vi "MGCC_MdlMgmt_Loads.vi"() -> ()   [LabVIEW 2016]
doc: "This VI is designed to initize the SHE215 model with loads (2D double array)."
uses:
  <vilib>/imath/engines/lvmath2/RunTimeEngine/NodeEndStatement/NIMS_NodeEndStatement_Output.vi
  <instcachedir>/0/NIMS_NodeEndStatement_Output_53EC0D466D134D7ABD903AC30B43404B.lvgen/NIMS_NodeEndStatement_Output_53EC0D466D134D7ABD903AC30B43404B_002.vi
  <vilib>/imath/engines/lvmath2/RunTimeEngine/ErrorHandling/NIMS_Finalize Error.vi
panel:
  out "array":dbl[][](array[numeric])
  out "text":string
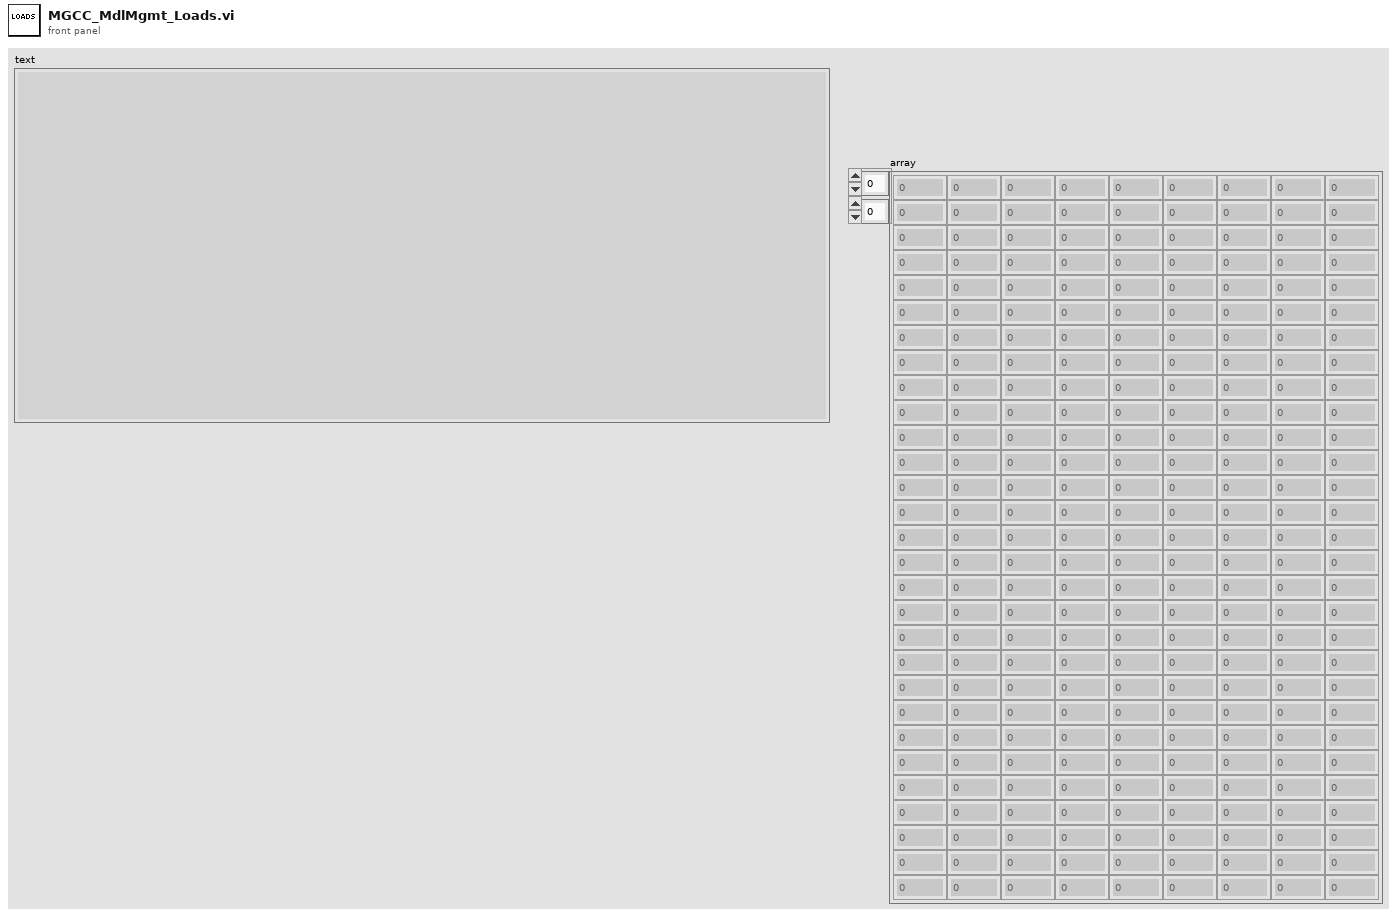
[diagram p1: front panel]
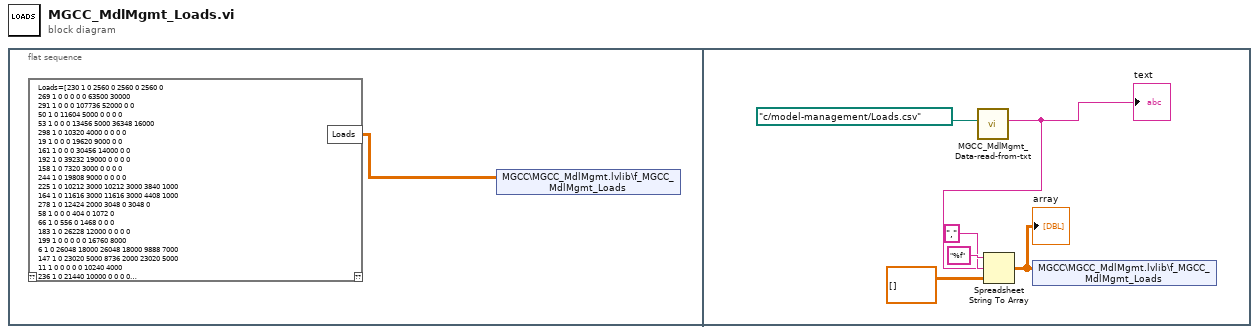
[diagram p0: block diagram]
diagram:
  n1 = flat-sequence {
    frame #0 {
      n2 = mathscript code="Loads=[230\t1\t0\t2560\t0\t2560\t0\t2560\t0\n269\t1\t0\t0\t0\t0\t0\t63500\t30000\n291\t1\t0\t0\t0\t107736\t52000\t0\t0\n50\t1\t0\t11604\t5000\t0\t0\t0\t0\n53\t1\t0\t0\t0\t13456\t5000\t36348\t16000\n298\t1\t0\t10320\t4000\t0\t0\t0\t0\n19\t1\t0\t0\t0\t19620\t9000\t0\t0\n161\t1\t0\t0\t0\t30456\t14000\t0\t0\n192\t1\t0\t39232\t19000\t0\t0\t0\t0\n158\t1\t0\t7320\t3000\t0\t0\t0\t0\n244\t1\t0\t19808\t9000\t0\t0\t0\t0\n225\t1\t0\t10212\t3000\t10212\t3000\t3840\t1000\n164\t1\t0\t11616\t3000\t11616\t3000\t4408\t1000\n278\t1\t0\t12424\t2000\t3048\t0\t3048\t0\n58\t1\t0\t0\t0\t404\t0\t1072\t0\n66\t1\t0\t556\t0\t1468\t0\t0\t0\n183\t1\t0\t26228\t12000\t0\t0\t0\t0\n199\t1\t0\t0\t0\t0\t0\t16760\t8000\n6\t1\t0\t26048\t18000\t26048\t18000\t9888\t7000\n147\t1\t0\t23020\t5000\t8736\t2000\t23020\t5000\n11\t1\t0\t0\t0\t0\t0\t10240\t4000\n236\t1\t0\t21440\t10000\t0\t0\t0\t0\n292\t1\t0\t0\t0\t7232\t3000\t0\t0\n163\t1\t0\t80516\t39000\t0\t0\t0\t0\n174\t1\t0\t33692\t16000\t0\t0\t0\t0\n133\t1\t0\t6412\t1000\t22208\t6000\t22208\t6000\n152\t1\t0\t1464\t0\t0\t0\t0\t0\n253\t1\t0\t10128\t5000\t26680\t13000\t26680\t13000\n218\t1\t0\t0\t0\t44332\t21000\t0\t0\n231\t1\t0\t0\t0\t0\t0\t47604\t23000\n61\t1\t0\t0\t0\t3384\t2000\t8948\t6000\n193\t1\t0\t0\t0\t60444\t29000\t0\t0\n207\t1\t0\t6444\t4000\t6444\t4000\t2404\t1000\n277\t1\t0\t32972\t15000\t0\t0\t0\t0\n57\t1\t0\t10560\t1000\t10560\t1000\t4008\t0\n17\t1\t0\t0\t0\t22604\t10000\t0\t0\n29\t1\t0\t0\t0\t0\t0\t12540\t6000\n22\t1\t0\t10916\t5000\t0\t0\t1732\t0\n166\t1\t0\t0\t0\t0\t0\t16996\t8000\n279\t1\t0\t22396\t3000\t22396\t3000\t22396\t3000\n224\t1\t0\t2932\t1000\t2932\t1000\t2932\t1000\n14\t1\t0\t2436\t0\t2436\t0\t924\t0\n123\t1\t0\t0\t0\t7226.66800000000\t5000\t7226.66800000000\t5000\n30\t1\t0\t0\t0\t12864\t6000\t0\t0\n280\t1\t0\t0\t0\t22808\t11000\t0\t0\n71\t1\t0\t0\t0\t0\t0\t17616\t8000\n167\t1\t0\t0\t0\t19296\t9000\t0\t0\n245\t1\t0\t0\t0\t0\t0\t26548\t12000\n246\t1\t0\t51136\t24000\t0\t0\t0\t0\n82\t1\t0\t2000\t1000\t2000\t1000\t2000\t1000\n2\t1\t0\t8008.00000000000\t2000\t8008.00000000000\t2000\t8008.00000000000\t2000\n266\t1\t0\t15176\t2000\t15176\t2000\t5720\t0\n191\t1\t0\t0\t0\t4188\t2000\t0\t0\n281\t1\t0\t11520\t3000\t11520\t3000\t11520\t3000\n222\t1\t0\t27944\t4000\t27944\t4000\t27944\t4000\n299\t1\t0\t0\t0\t0\t0\t57232\t27000\n142\t1\t0\t0\t0\t0\t0\t39868\t19000\n52\t1\t0\t0\t0\t0\t0\t34656\t16000\n295\t1\t0\t37948\t18000\t0\t0\t0\t0\n77\t1\t0\t9404\t2000\t24780\t7000\t24780\t7000\n284\t1\t0\t0\t0\t876\t0\t2312\t0\n28\t1\t0\t0\t0\t0\t0\t12292\t5000\n188\t1\t0\t19256\t9000\t0\t0\t0\t0\n78\t1\t0\t746.668000000000\t0\t746.668000000000\t0\t746.668000000000\t0\n223\t1\t0\t0\t0\t0\t0\t42192\t20000\n39\t1\t0\t17600\t8000\t0\t0\t0\t0\n283\t1\t0\t32996\t14000\t32996\t14000\t32996\t14000\n81\t1\t0\t0\t0\t0\t0\t32980\t15000\n238\t1\t0\t43344\t21000\t0\t0\t0\t0\n153\t1\t0\t9200\t4000\t9200\t4000\t9200\t4000\n160\t1\t0\t900\t0\t0\t0\t0\t0\n184\t1\t0\t0\t0\t0\t0\t20420\t9000\n293\t1\t0\t10452\t4000\t10452\t4000\t10452\t4000\n141\t1\t0\t4320\t2000\t0\t0\t0\t0\n5\t1\t0\t0\t0\t0\t0\t10212\t4000\n262\t1\t0\t4360\t0\t4360\t0\t4360\t0\n237\t1\t0\t0\t0\t8560\t4000\t0\t0\n121\t1\t0\t0\t0\t43704\t21000\t0\t0\n228\t1\t0\t45936\t22000\t7320\t3000\t7320\t3000\n101\t1\t0\t0\t0\t0\t0\t63344\t30000\n255\t1\t0\t0\t0\t0\t0\t59820\t28000\n104\t1\t0\t9944\t3000\t0\t0\t3760\t1000\n210\t1\t0\t27556\t13000\t0\t0\t0\t0\n263\t1\t0\t26292\t9000\t26292\t9000\t6440\t1000\n221\t1\t0\t22576\t10000\t22576\t10000\t420\t0\n33\t1\t0\t1324\t0\t1324\t0\t1324\t0\n242\t1\t0\t1068\t0\t1068\t0\t1068\t0\n235\t1\t0\t17704\t1000\t17704\t1000\t17704\t1000\n240\t1\t0\t0\t0\t0\t0\t18944\t9000\n226\t1\t0\t20084\t3000\t20084\t3000\t20084\t3000\n270\t1\t0\t7056\t3000\t156\t0\t0\t0\n72\t1\t0\t14688\t7000\t0\t0\t0\t0\n258\t1\t0\t0\t0\t0\t0\t50752\t24000\n75\t1\t0\t928\t0\t0\t0\t0\t0\n243\t1\t0\t0\t0\t0\t0\t16256\t7000\n286\t1\t0\t3840\t1000\t0\t0\t0\t0\n256\t1\t0\t9332\t2000\t9332\t2000\t9332\t2000\n48\t1\t0\t16212\t3000\t16212\t3000\t16212\t3000\n135\t1\t0\t22012\t10000\t0\t0\t0\t0\n143\t1\t0\t640\t0\t1688\t1000\t1688\t1000\n190\t1\t0\t0\t0\t0\t0\t8088.00000000000\t3000\n220\t1\t0\t0\t0\t0\t0\t2048\t0\n124\t1\t0\t0\t0\t5192\t2000\t0\t0\n95\t1\t0\t640\t0\t1688\t1000\t1688\t1000\n211\t1\t0\t0\t0\t10860\t5000\t0\t0\n213\t1\t0\t19744\t9000\t0\t0\t0\t0\n289\t1\t0\t13120\t4000\t13120\t4000\t13120\t4000\n296\t1\t0\t0\t0\t0\t0\t26912\t13000\n185\t1\t0\t4716\t1000\t4716\t1000\t1792\t0\n45\t1\t0\t1920\t2000\t1920\t2000\t1920\t2000\n249\t1\t0\t0\t0\t2960\t0\t7960\t1000\n271\t1\t0\t15572\t3000\t15572\t3000\t15572\t3000\n54\t1\t0\t11652\t5000\t0\t0\t0\t0\n180\t1\t0\t0\t0\t0\t0\t57236\t27000\n251\t1\t0\t36360\t17000\t0\t0\t0\t0\n265\t1\t0\t83860\t14000\t83860\t14000\t83860\t14000\n227\t1\t0\t2432\t1000\t9216\t4000\t9216\t4000\n282\t1\t0\t9064\t3000\t9064\t3000\t9064\t3000\n259\t1\t0\t0\t0\t3908\t1000\t0\t0\n51\t1\t0\t22808\t11000\t0\t0\t0\t0\n294\t1\t0\t16852\t7000\t16852\t7000\t16852\t7000\n268\t1\t0\t0\t0\t0\t0\t33892\t16000\n115\t1\t0\t0\t0\t76\t0\t0\t0\n288\t1\t0\t103456\t33000\t103456\t33000\t103456\t33000\n155\t1\t0\t4864\t2000\t0\t0\t0\t0\n287\t1\t0\t62856\t30000\t0\t0\t0\t0\n70\t1\t0\t0\t0\t33960\t16000\t0\t0\n168\t1\t0\t3632\t0\t3632\t0\t17744\t4000\n241\t1\t0\t852\t0\t0\t0\t0\t0\n165\t1\t0\t0\t0\t10044\t4000\t0\t0\n254\t1\t0\t0\t0\t616\t0\t0\t0\n234\t1\t0\t1600\t0\t1600\t0\t1600\t0\n195\t1\t0\t0\t0\t34356\t16000\t0\t0\n47\t1\t0\t0\t0\t0\t0\t408\t0\n10\t1\t0\t0\t0\t5316\t2000\t14056\t5000\n208\t1\t0\t12160\t5000\t0\t0\t0\t0\n202\t1\t0\t0\t0\t0\t0\t31764\t15000\n179\t1\t0\t0\t0\t7380\t0\t28308\t7000\n267\t1\t0\t76364\t0\t76364\t0\t76364\t0\n248\t1\t0\t3732\t1000\t3732\t1000\t3732\t1000\n276\t1\t0\t21384\t3000\t21384\t3000\t21384\t3000\n297\t1\t0\t12888\t2000\t12888\t2000\t12888\t2000\n216\t1\t0\t720\t0\t720\t0\t720\t0\n219\t1\t0\t0\t0\t0\t0\t67472\t32000\n9\t1\t0\t0\t0\t21872\t9000\t2452\t0\n114\t1\t0\t13568\t0\t5132\t0\t0\t0\n84\t1\t0\t6480\t3000\t0\t0\t0\t0\n131\t1\t0\t0\t0\t0\t0\t11040\t5000];"() -> ("Loads"=w1:dbl[][])  [unwired: 1 in, 1 out]
      n3 = shared-variable "MGCC\\MGCC_MdlMgmt.lvlib\\f_MGCC_MdlMgmt_Loads"(w1) -> ()  [unwired: 1 in, 1 out]
    }
    frame #1 {
      n4 = call "MGCC_MdlMgmt_Data-read-from-txt.vi"("file path (use dialog)"=path "c:/model-management/Loads.csv") -> ("text"=w15:string)  [unwired: 10 in]
      "text" <- w15
      n5 = Spreadsheet String To Array(delimiter (Tab)=",", format string="%f", spreadsheet string=w15, array type (2D Dbl)=dbl[][] []) -> (array=w16:dbl[][])
      "array" <- w16
      n6 = shared-variable "MGCC\\MGCC_MdlMgmt.lvlib\\f_MGCC_MdlMgmt_Loads"(w16) -> ()  [unwired: 1 in, 1 out]
    }
  }
